vi "rqcBob Operation Mode.vi"(0 "rqcBob in":refnum<class "rqcBob.lvclass">, 5 "Operation Mode":T1=enum."Channel Test", 11 "error in (no error)":errorcluster) -> (4 "rqcBob out":refnum<class "rqcBob.lvclass">, 15 "error out":errorcluster)   [LabVIEW 2018, in "rqcBob.lvclass"]
uses:
  rqcBob.lvclass
  Custom Controls/rqcBob Operation Mode.ctl
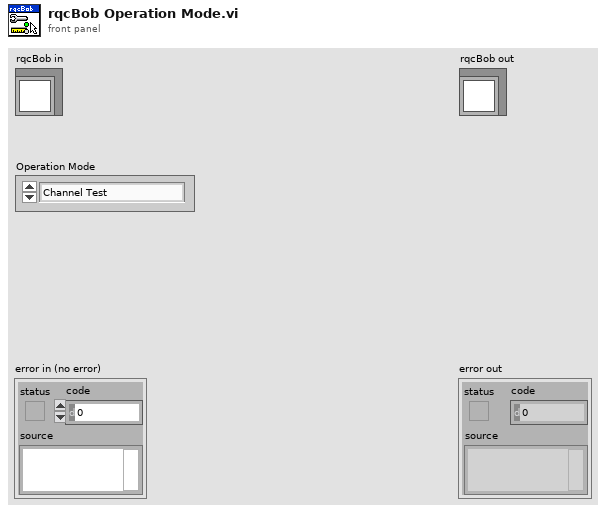
[diagram p1: front panel]
types:
  T1 = typedef "rqcBob.lvclass/rqcBob Operation Mode.ctl" = enum16{"Not Set", "Channel Test", "Key Distribution", "Modulation Level Test", "Window Test", "Delay Line Test", "Alice Modulation Level Test"}
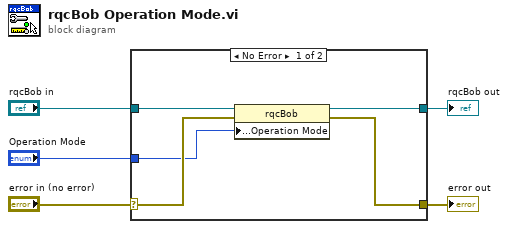
[diagram p0: block diagram]
diagram:
  n1 = case shown="No Error" "error in (no error)" {
    selector: "error in (no error)" -> [w8 w12]
    tunnel: [w7 w12] -> w4
    tunnel: [w9 w11] -> w2
    tunnel: "rqcBob in" -> [w10 w11]
    tunnel: "Operation Mode" -> [w6 _]
    frame No Error {
      n2 = property class="rqcBob"(reference=w10, error in=w8, "public:Public Properties Access:Operation Mode"=w6) -> (reference out=w9:refnum<class "rqcBob.lvclass">, error out=w7:errorcluster)
    }
    frame Error {
    }
  }
  "error out" <- w4
  "rqcBob out" <- w2
